vi "labview_test.vi"() -> ()   [LabVIEW 2021]
uses:
  <vilib>/Utility/file.llb/Read Delimited Spreadsheet (DBL).vi
  <vilib>/Analysis/Matrix/Numeric/Conversions/Array To Matrix - RA2.vi
  <vilib>/Analysis/Matrix/Numeric/Conversions/Matrix To Array - CM.vi
  <vilib>/Analysis/Matrix/NI_Matrix.lvlib
panel:
  out "LabVIEWEigenvectors":cdb[][](array[numeric])
  out "LabveiwEigenvalues":cdb[](array[numeric])
  out "Elapsed time":dbl=0.5790897820043028
  out "ScipyEigenvectors":dbl[][](array[numeric])
  out "ScipyEigenvalues":dbl[](array[numeric])
  out "standard output":string
  out "standard error":string
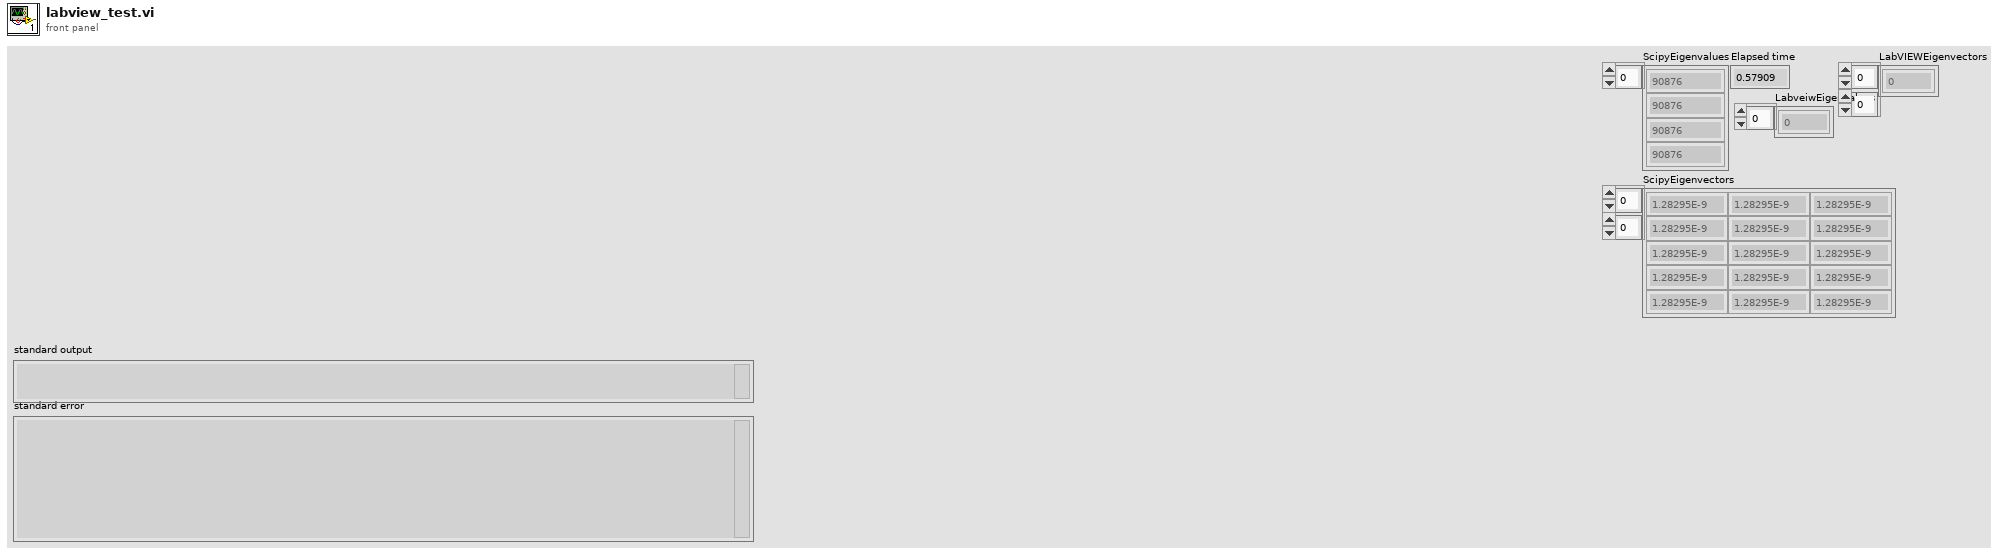
[diagram p1: front panel]
types:
  T1 = typedef "NI_Matrix.lvlib/RealMatrix.ctl" = dbl[][]
  T2 = typedef "NI_Matrix.lvlib/ComplexMatrix.ctl" = cdb[][]
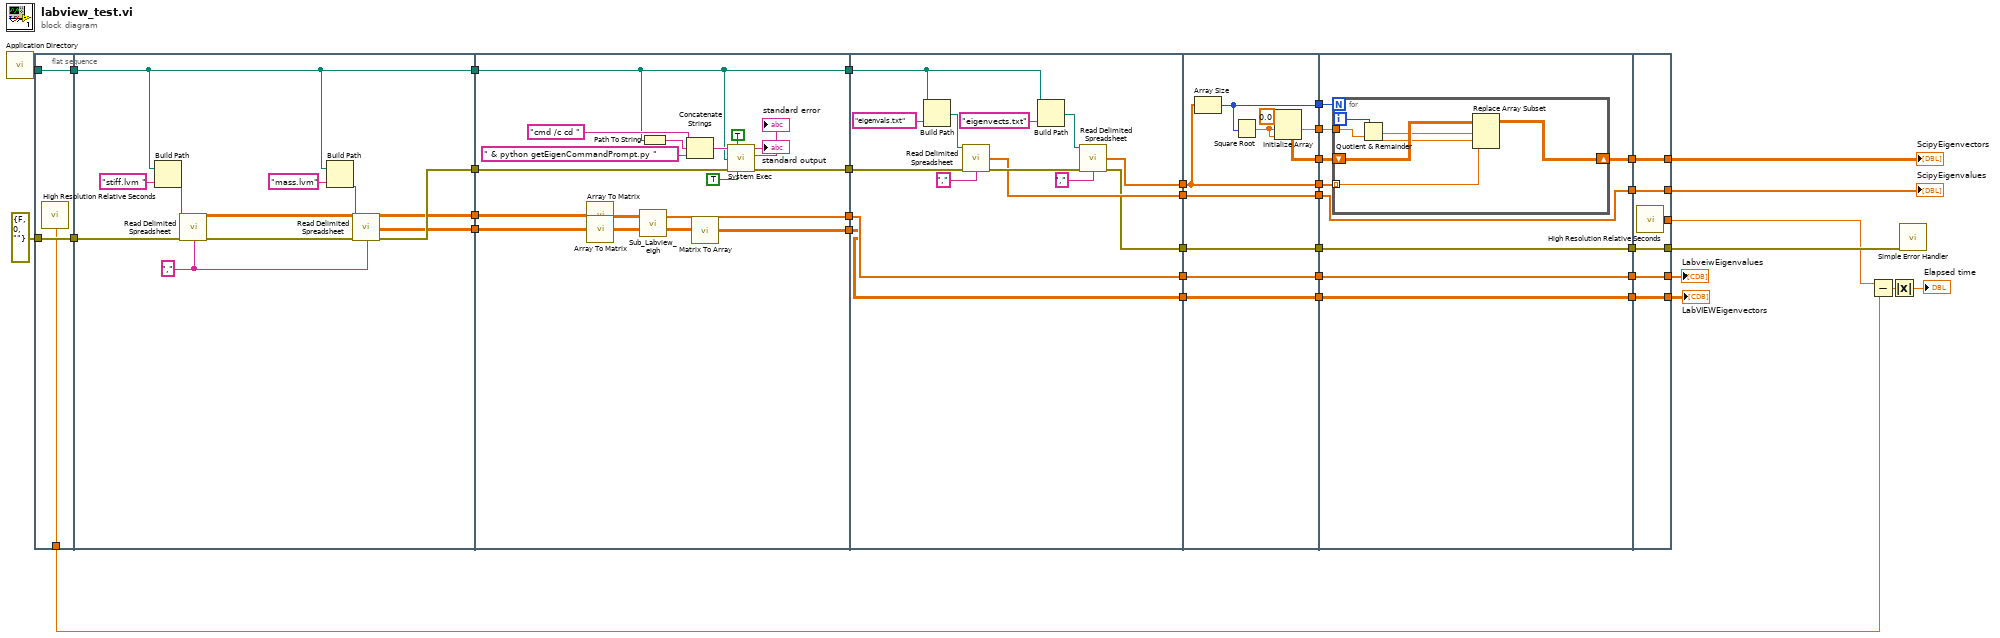
[diagram p0: block diagram]
diagram:
  n1 = call <vilib>:"Application Directory.vi"() -> ("Application Directory"=w25:path)
  n2 = flat-sequence {
    tunnel: errorcluster {"status"=FALSE, "code"=0, "source"=""} ("error in (no error)") -> [w41]
    tunnel: w25 -> [w42]
    tunnel: [w42] -> w15
    tunnel: [w41] -> w16
    tunnel: [w40] -> w19
    tunnel: w16 -> [w46]
    tunnel: w15 -> [w51]
    tunnel: [w51] -> w14
    tunnel: [w45] -> w13
    tunnel: [w44] -> w12
    tunnel: [w43] -> w11
    tunnel: [w69] -> w39
    tunnel: w14 -> [w63]
    tunnel: [w63] -> w38
    tunnel: w13 -> [w70]
    tunnel: w12 -> [w59]
    tunnel: w11 -> [w60]
    tunnel: [w55] -> w10
    tunnel: [w54] -> w9
    tunnel: w39 -> [w85]
    tunnel: w38 -> [w83]
    tunnel: [w78] -> w37
    tunnel: [w77] -> w36
    tunnel: [w74] -> w35
    tunnel: w10 -> [w73]
    tunnel: w9 -> [w72]
    tunnel: [w73] -> w8
    tunnel: [w72] -> w7
    tunnel: w37 -> [w89]
    tunnel: w36 -> [w91]
    tunnel: [w94] -> w34
    tunnel: [w92] -> w33
    tunnel: [w91] -> w32
    tunnel: [w90] -> w31
    tunnel: [w89] -> w30
    tunnel: w35 -> [w88]
    tunnel: [w88] -> w29
    tunnel: w8 -> [w86]
    tunnel: w7 -> [w87]
    tunnel: [w87] -> w6
    tunnel: [w86] -> w3
    tunnel: w34 -> [w103]
    tunnel: w33 -> [w102]
    tunnel: w32 -> [w101]
    tunnel: w31 -> [w100]
    tunnel: w30 -> [w98]
    tunnel: w29 -> [w97]
    tunnel: [w99] -> w28
    tunnel: [w98] -> w27
    tunnel: [w97] -> w26
    tunnel: w6 -> [w96]
    tunnel: [w96] -> w5
    tunnel: [w95] -> w4
    tunnel: w3 -> [w95]
    tunnel: w28 -> [w116]
    tunnel: w27 -> [w115]
    tunnel: w26 -> [w114]
    tunnel: [w116] -> w22
    tunnel: [w115] -> w23
    tunnel: [w114] -> w21
    tunnel: [w113] -> w20
    tunnel: [w112] -> w1
    tunnel: w5 -> [w112]
    tunnel: w4 -> [w111]
    tunnel: [w111] -> w2
    frame #0 {
      n3 = call <vilib>:"High Resolution Relative Seconds.vi"() -> ("relative seconds"=w40:dbl)
    }
    frame #1 {
      w48 = "," ("delimiter (\\t)")
      n4 = Build Path(base path=w51, name or relative path="stiff.lvm ") -> (appended path=w50:path)
      n5 = call-poly <vilib>:"Read Delimited Spreadsheet.vi"("file path (dialog if empty)"=w50, "error in (no error)"=w46, "delimiter (\\t)"=w48) -> ("all rows"=w43:dbl[][], "error out"=w47:errorcluster)  [unwired: 7 in, 4 out]
      n6 = Build Path(base path=w51, name or relative path="mass.lvm") -> (appended path=w49:path)
      n7 = call-poly <vilib>:"Read Delimited Spreadsheet.vi"("file path (dialog if empty)"=w49, "error in (no error)"=w47, "delimiter (\\t)"=w48) -> ("all rows"=w44:dbl[][], "error out"=w45:errorcluster)  [unwired: 7 in, 4 out]
    }
    frame #2 {
      n8 = call-poly <vilib>:"Array To Matrix.vi"("Real 2D Array"=w60) -> ("Real Matrix"=w57:T1)
      n9 = call-poly <vilib>:"Array To Matrix.vi"("Real 2D Array"=w59) -> ("Real Matrix"=w58:T1)
      n10 = call "Sub_Labview_eigh.vi"("Mass"=w58, "Stiffness"=w57) -> ("Eigenvectors"=w56:T2, "Eigenvalues"=w55:cdb[])
      n11 = Path To String(path=w63) -> (string=w62:string)
      n12 = Concatenate Strings("cmd /c cd " ("command line"), w62, " & python getEigenCommandPrompt.py " ("standard input")) -> (w64:string)
      n13 = call-poly <vilib>:"Matrix To Array.vi"("Complex Matrix"=w56) -> ("Complex 2D Array"=w54:cdb[][])
      n14 = call <vilib>:"System Exec.vi"("run minimized? (F)"=TRUE, "wait until completion? (T)"=TRUE, "error in (no error)"=w70, "working directory"=w63, "command line"=w64) -> ("error out"=w69:errorcluster, "standard error"=→"standard error":string, "standard output"=→"standard output":string)  [unwired: 3 in, 1 out]
    }
    frame #3 {
      n15 = Build Path(base path=w83, name or relative path="eigenvals.txt") -> (appended path=w82:path)
      n16 = call-poly <vilib>:"Read Delimited Spreadsheet.vi"("file path (dialog if empty)"=w82, "error in (no error)"=w85, "delimiter (\\t)"="," ("delimiter (\\t)")) -> ("first row"=w78:dbl[], "error out"=w84:errorcluster)  [unwired: 7 in, 4 out]
      n17 = Build Path(base path=w83, name or relative path="eigenvects.txt") -> (appended path=w81:path)
      n18 = call-poly <vilib>:"Read Delimited Spreadsheet.vi"("file path (dialog if empty)"=w81, "error in (no error)"=w84, "delimiter (\\t)"="," ("delimiter (\\t)")) -> ("first row"=w77:dbl[], "error out"=w74:errorcluster)  [unwired: 7 in, 4 out]
    }
    frame #4 {
      n19 = Array Size(array=w91) -> (size(s)=w94:i32)
      n20 = Square Root(x=w94) -> (sqrt(x)=w90:dbl)
      n21 = Initialize Array(0.0 ("element"), w90, w90) -> (w92:dbl[][])
    }
    frame #5 {
      n22 = for {
        N: w103 -> [_]
        shift-right: [w106] -> w99
        shift-left: w102 -> [w109]
        tunnel: w101 -> [w108] mode=indexing
        tunnel: w100 -> [w105]
        i -> [w110]
        n23 = Quotient & Remainder(x=w110, y=w105) -> (x-y*floor(x/y)=w104:dbl, floor(x/y)=w107:dbl)
        n24 = Replace Array Subset(array=w109, new element=w108, index (row)=w107, index (col)=w104) -> (w106:dbl[][])
      }
    }
    frame #6 {
      n25 = call <vilib>:"High Resolution Relative Seconds.vi"() -> ("relative seconds"=w113:dbl)
    }
  }
  n26 = Subtract(x=w20, y=w19) -> (x-y=w18:dbl)
  n27 = Absolute Value(x=w18) -> (abs(x)=→"Elapsed time":dbl)
  n28 = call <vilib>:"Simple Error Handler.vi"("error in (no error)"=w21) -> ()  [unwired: 4 in, 5 out]
  "ScipyEigenvalues" <- w23
  "ScipyEigenvectors" <- w22
  "LabveiwEigenvalues" <- w2
  "LabVIEWEigenvectors" <- w1
